vi "BuildMessage.vi"(7 "generate_outcome":bool, 8 "error in":errorcluster, 11 "Image":T1) -> (0 "error out":errorcluster, 2 "JSON string":string, 3 "Image Out (duplicate)":T1)   [LabVIEW 2019]
uses:
  <vilib>/vision/Image Controls.llb/IMAQ Image.ctl
  RecognitionRequest.ctl
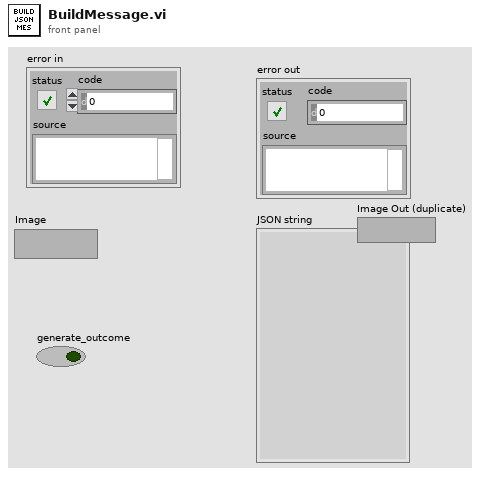
[diagram p1: front panel]
types:
  T1 = typedef "IMAQ Image.ctl" = refnum<image>
  T2 = typedef "RecognitionRequest.ctl" = cluster{"generate_outcome":bool, "detection_location":string, "agent_name":string, "face_image":string, "base64encoded":bool}
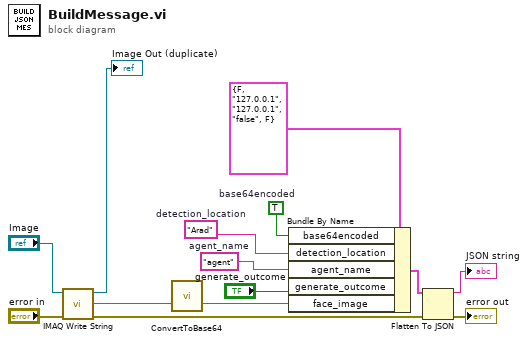
[diagram p0: block diagram]
diagram:
  w2 = TRUE  # base64encoded
  w13 = "Arad"  # detection_location
  w14 = "agent"  # agent_name
  n1 = call-poly "IMAQ Write String"("error in (no error)"="error in", "Image"="Image") -> ("error out"=w10:errorcluster, "FileString"=w4:string, "Image Out (duplicate)"=→"Image Out (duplicate)":T1)  [unwired: 7 in]
  n2 = call "ConvertToBase64.vi"("String"=w4) -> ("Base64 String"=w3:string)  [unwired: 10 in]
  n3 = Bundle By Name(cluster=T2 {"generate_outcome"=FALSE, "detection_location"="127.0.0.1", "agent_name"="127.0.0.1", "face_image"="false", "base64encoded"=FALSE} ("RecognitionRequest"), "base64encoded"=w2, "detection_location"=w13, "agent_name"=w14, "generate_outcome"="generate_outcome", "face_image"=w3) -> (w12:T2)
  n4 = Flatten To JSON(anything=w12, error in (no error)=w10) -> (JSON string=→"JSON string":string, 11:→"error out":errorcluster)  [unwired: 1 in]
